vi "CreateQueueMessage.vi"(5 "elements to preallocate (0)":i32, 6 "create if not found? (T)":bool=TRUE, 7 "max queue size (-1, unlimited)":i32=-1, 8 "error in":errorcluster, 9 "initial message data []":variant[](array[variant]), 10 "initial message names []":string[](array[string]), 11 "name (\"\", unnamed)":string) -> (0 "error out":errorcluster, 1 "elements preallocated":i32, 3 "message ref":refnum<class "CLM_LocalMessage_Queue.lvclass">, 4 "created new?":bool)   [LabVIEW 2013, in "CLM_LocalMessage_Queue.lvclass"]
uses:
  CLM_LocalMessage_Queue.lvclass
  LocalMessage/Message.ctl
  CLM_LocalMessage_Queue.lvclass/CLM_LocalMessage_Queue.ctl
  SendQueueMessage.vi
  SendQueueMessage_Cluster.vi
  LocalMessage/BundleMessageCluster.vi
  LocalMessage/CLM_LocalMessage.lvclass
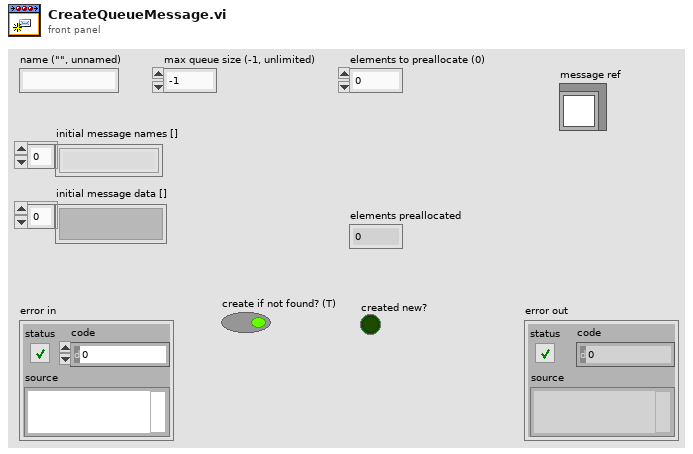
[diagram p1: front panel]
types:
  T1 = typedef "CLM_LocalMessage.lvclass/Message.ctl" = cluster{"name":string, "data":variant, "attributes":variant, "urgent":bool}
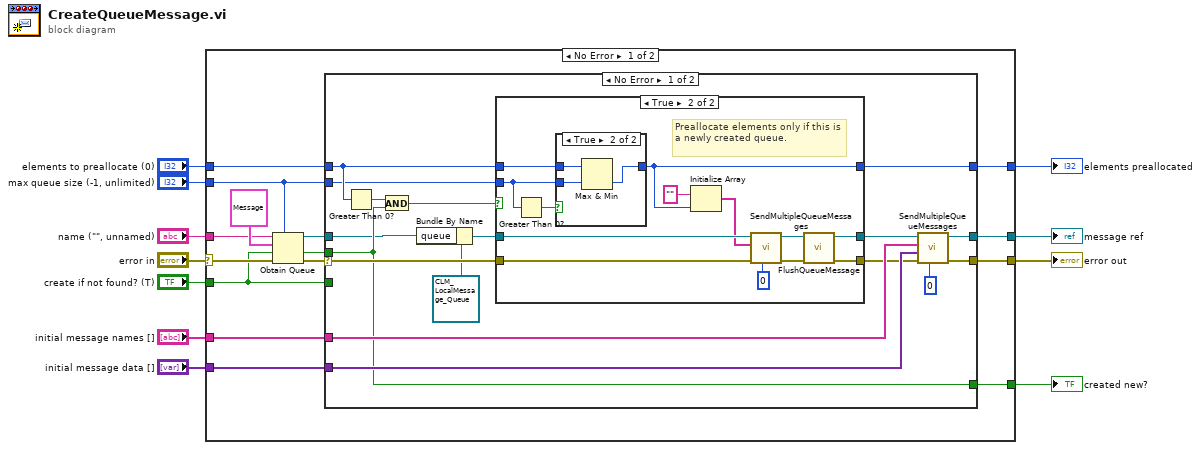
[diagram p0: block diagram]
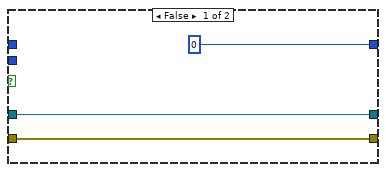
[diagram p2: hidden frame]
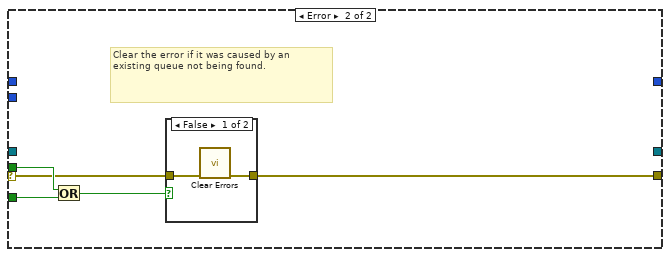
[diagram p4: hidden frame]
diagram:
  n1 = case shown="No Error" "error in" {
    selector: "error in" -> [w26 w72]
    tunnel: "name (\"\", unnamed)" -> [w24 _]
    tunnel: "initial message names []" -> [w23 _]
    tunnel: "initial message data []" -> [w22 _]
    tunnel: [w21 w72] -> w7
    tunnel: [w20 _] -> w6
    tunnel: [w13 _] -> w5
    tunnel: "elements to preallocate (0)" -> [w17 _]
    tunnel: "max queue size (-1, unlimited)" -> [w16 _]
    tunnel: [w15 _] -> w2
    tunnel: "create if not found? (T)" -> [w12 _]
    frame No Error {
      n2 = Obtain Queue(max queue size (-1, unlimited)=w16, name (unnamed)=w24, element data type=T1 {"name"="", "data"=variant, "attributes"=variant, "urgent"=FALSE} ("message"), create if not found? (T)=w12, error in (no error)=w26) -> (queue out=w19:refnum<queue>, created new?=w18:bool, error out=w14:errorcluster)
      n3 = case shown="No Error" w14 {
        selector: w14 -> [w32 w65]
        tunnel: w23 -> [w43 _]
        tunnel: w22 -> [w42 _]
        tunnel: [w40 w64] -> w21
        tunnel: [w30 _] -> w20
        tunnel: w19 -> [w28 _]
        tunnel: w18 -> [w31 w67]
        tunnel: w17 -> [w35 _]
        tunnel: w16 -> [w34 _]
        tunnel: [w33 _] -> w15
        tunnel: [w31 _] -> w13
        tunnel: w12 -> [_ w68]
        frame No Error {
          n4 = Greater Than 0?(x=w35) -> (x > 0?=w37:bool)
          n5 = And(x=w37, y=w31) -> (x .and. y?=w36:bool)
          n6 = Bundle By Name(cluster=refnum<class "CLM_LocalMessage_Queue.lvclass"> refnum ("CLM_LocalMessage_Queue.lvclass"), "queue"=w28) -> (w27:refnum<class "CLM_LocalMessage_Queue.lvclass">)
          n7 = case shown="True" w36 {
            tunnel: w27 -> [w46 w59]
            tunnel: [w46 w52] -> w39
            tunnel: w32 -> [w45 w58]
            tunnel: [w45 w51] -> w38
            tunnel: w35 -> [_ w48]
            tunnel: w34 -> [_ w49]
            tunnel: [0 ("elements to preallocate (0)") w47] -> w33
            frame False {
            }
            frame True {
              # "Preallocate elements only if this is a newly created queue."
              n8 = Greater Than 0?(x=w49) -> (x > 0?=w50:bool)
              n9 = case shown="True" w50 {
                tunnel: w49 -> [_ w62]
                tunnel: w48 -> [w60 w63]
                tunnel: [w60 w61] -> w47
                frame False {
                }
                frame True {
                  n10 = Max & Min(x=w63, y=w62) -> (min(x,y)=w61:i32)  [unwired: 1 out]
                }
              }
              n11 = Initialize Array("", w47) -> (w55:string[])
              n12 = call "SendMultipleQueueMessages.vi"("timeout in ms (-1)"=0, "error in"=w58, "message names []"=w55, "message ref in"=w59) -> ("error out"=w53:errorcluster, "message ref out"=w54:refnum<class "CLM_LocalMessage_Queue.lvclass">)  [unwired: 5 in, 1 out]
              n13 = call "FlushQueueMessage.vi"("error in"=w53, "message ref in"=w54) -> ("error out"=w51:errorcluster, "message ref out out"=w52:refnum<class "CLM_LocalMessage_Queue.lvclass">)  [unwired: 7 in, 1 out]
            }
          }
          n14 = call "SendMultipleQueueMessages.vi"("timeout in ms (-1)"=0, "error in"=w38, "message data []"=w42, "message names []"=w43, "message ref in"=w39) -> ("error out"=w40:errorcluster, "message ref out"=w30:refnum<class "CLM_LocalMessage_Queue.lvclass">)  [unwired: 4 in, 1 out]
        }
        frame Error {
          # "Clear the error if it was caused by an existing queue not being found."
          n15 = Or(x=w67, y=w68) -> (x .or. y?=w66:bool)
          n16 = case shown="False" w66 {
            tunnel: w65 -> [w70 w71]
            tunnel: [w69 w71] -> w64
            frame False {
              n17 = call <vilib>:"Clear Errors.vi"("error in (no error)"=w70) -> ("error out"=w69:errorcluster)  [unwired: 6 in]
            }
            frame True {
            }
          }
        }
      }
    }
    frame Error {
    }
  }
  "error out" <- w7
  "message ref" <- w6
  "elements preallocated" <- w2
  "created new?" <- w5
